vi "LAX100.vi"() -> ()   [LabVIEW 2015]
uses:
  <vilib>/Instr/_visa.llb/VISA Configure Serial Port (Instr).vi
panel:
  out "Serial Settings:Number of Bytes at Serial Port":u32
  out "error out 4":errorcluster
  out "error out":errorcluster
  out "error out 3":errorcluster
  out "VISA resource name out":refnum<visa-resource-name>
  in  "error out 2":errorcluster
  out "read buffer":string
  in  "stop":bool
  out "CMD":string
  in  "shutter":bool
  in  "power":bool
  in  "Intensity":dbl
  # "LAX-C100"
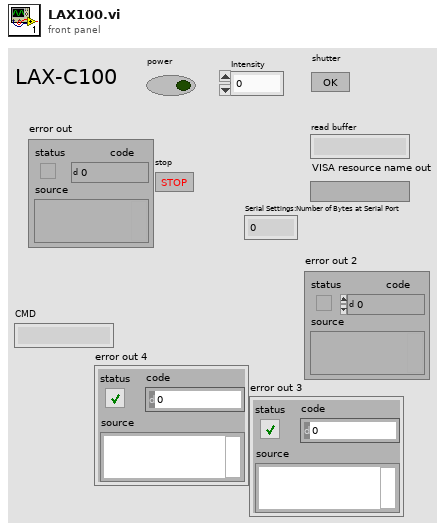
[diagram p1: front panel]
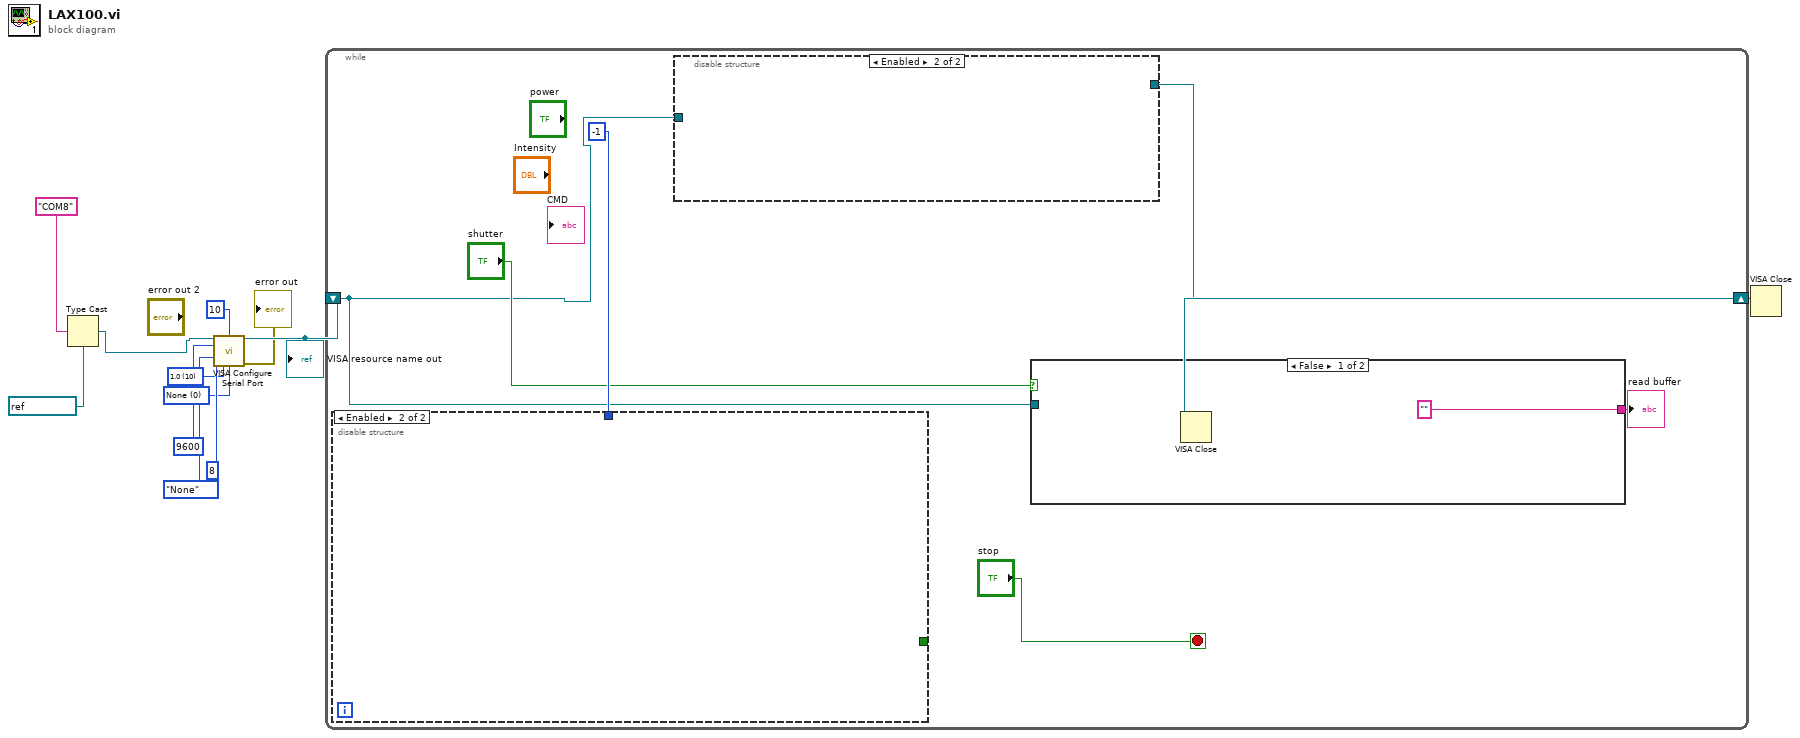
[diagram p0: block diagram]
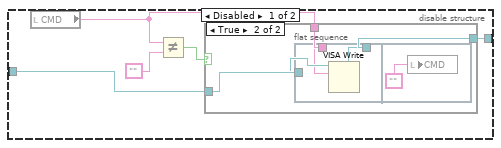
[diagram p2: hidden frame]
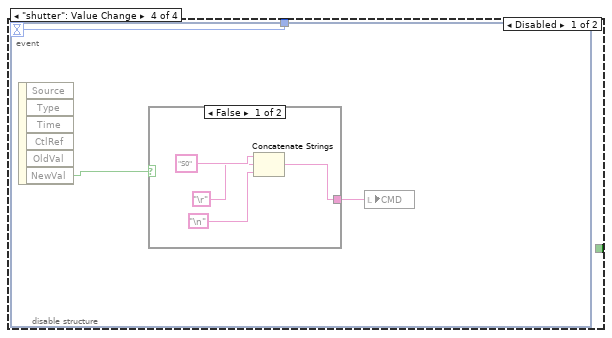
[diagram p4: hidden frame]
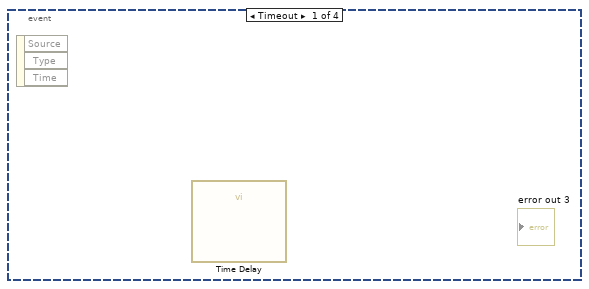
[diagram p5: hidden frame]
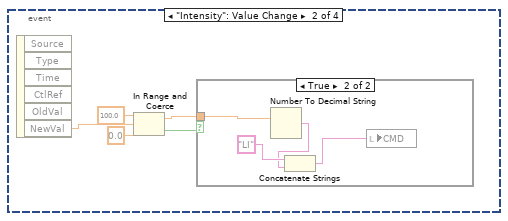
[diagram p6: hidden frame]
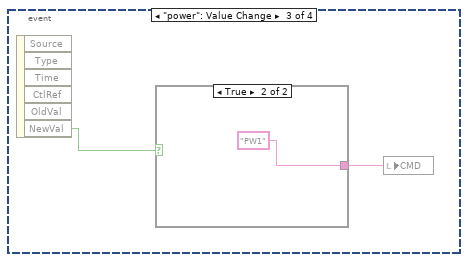
[diagram p8: hidden frame]
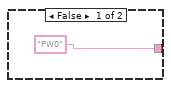
[diagram p9: hidden frame]
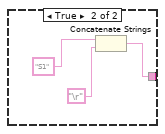
[diagram p10: hidden frame]
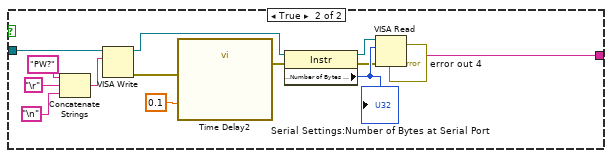
[diagram p11: hidden frame]
diagram:
  w6 = u16 0 items=["None", "XON/XOFF", "RTS/CTS", "XON/XOFF & RTS/CTS", "DTR/DSR", "XON/XOFF & DTR/DSR"] ("flow control (0:none)")
  w7 = u16 10 items=["1.0"=10, "1.5"=15, "2.0"=20] ("stop bits (10: 1 bit)")
  n1 = Type Cast(type=refnum<visa-resource-name> "COM12" ("VISA resource name"), x="COM8") -> (*(type *) &x=w2:refnum<visa-resource-name>)
  n2 = call-poly "VISA Configure Serial Port"("VISA resource name"=w2, "termination char\n(0xA = '\\n' = LF)"=u8 10 ("termination char\n(0xA = '\\n' = LF)"), "baud rate (9600)"=u32 9600, "data bits (8)"=u16 8, "parity (0:none)"=enum16{"None", "Odd", "Even", "Mark", "Space"}."None", "stop bits (10: 1 bit)"=w7, "flow control (0:none)"=w6) -> ("VISA resource name out"=w9:refnum<visa-resource-name>, "error out"=→"error out":errorcluster)  [unwired: 7 in]
  "VISA resource name out" <- w9
  n3 = while {
    shift-right: [w17] -> w8
    shift-left: w9 -> [w15]
    stop <- "stop" stop-if-true
    n4 = disable-structure shown="Enabled" {
      disable-tunnel: _ -> [w32 _]
      disable-tunnel: -1 -> [w31 _]
      frame Disabled {
        n5 = event shown="[3] \"shutter\": Value Change" {
          selector: _ -> [_ _ _ _]
          dyn-events: _ -> [_ _ _ _]
          timeout: w31 -> [_ _ _ _]
          event Timeout {
            n6 = event-data() -> ()  [unwired: 1 in, 3 out]
            n7 = call "Time Delay"() -> ()  [unwired: 11 in, 1 out]
          }
          event "Intensity": Value Change {
            n8 = event-data() -> ("NewVal"=w37:dbl)  [unwired: 1 in, 5 out]
            n9 = In Range and Coerce(upper limit=100.0, x=w37, lower limit=0.0) -> (coerced(x)=w33:dbl, In Range?=w34:bool)
            n10 = case shown="True" w34 {
              tunnel: w33 -> [_ w41]
              frame False {
              }
              frame True {
                n11 = Number To Decimal String(number=w41) -> (decimal integer string=w39:string)  [unwired: 1 in]
                n12 = Concatenate Strings("LI", w39) -> (w38:string)
                n13 = local write "CMD"(w38) -> ()
              }
            }
          }
          event "power": Value Change {
            n14 = event-data() -> ("NewVal"=w43:bool)  [unwired: 1 in, 5 out]
            n15 = case shown="True" w43 {
              tunnel: ["PW0" "PW1"] -> w42
              frame False {
              }
              frame True {
              }
            }
            n16 = local write "CMD"(w42) -> ()
          }
          event "shutter": Value Change {
            n17 = event-data() -> ("NewVal"=w47:bool)  [unwired: 1 in, 5 out]
            n18 = case shown="False" w47 {
              tunnel: [w50 w52] -> w46
              frame False {
                n19 = Concatenate Strings("S0", "\r", "\n") -> (w50:string)
              }
              frame True {
                n20 = Concatenate Strings("S1", "\r") -> (w52:string)
              }
            }
            n21 = local write "CMD"(w46) -> ()
          }
        }
      }
      frame Enabled {
      }
    }
    n22 = disable-structure shown="Enabled" {
      disable-tunnel: [w20 _] -> w17
      disable-tunnel: w15 -> [w19 _]
      frame Disabled {
        n23 = local read "CMD"() -> (w23:string)
        n24 = Not Equal?(x=w23, y="") -> (x != y?=w22:bool)
        n25 = case shown="True" w22 {
          tunnel: [_ w26] -> w20
          tunnel: w23 -> [_ w25]
          tunnel: w19 -> [_ w24]
          frame False {
          }
          frame True {
            n26 = flat-sequence {
              tunnel: [w29] -> w26
              tunnel: w24 -> [w28]
              tunnel: w25 -> [w27]
              frame #0 {
                n27 = VISA Write(VISA resource name=w28, write buffer=w27) -> (VISA resource name out=w29:refnum<visa-resource-name>)  [unwired: 1 in, 2 out]
              }
              frame #1 {
                n28 = local write "CMD"("") -> ()
              }
            }
          }
        }
      }
      frame Enabled {
      }
    }
    n29 = case shown="False" "shutter" {
      tunnel: w15 -> [_ w66]
      tunnel: ["" ("read buffer") w58] -> w14
      frame False {
      }
      frame True {
        n30 = Concatenate Strings("PW?", "\r", "\n") -> (w67:string)
        n31 = VISA Write(VISA resource name=w66, write buffer=w67) -> (VISA resource name out=w62:refnum<visa-resource-name>, error out=w65:errorcluster)  [unwired: 1 in, 1 out]
        n32 = call "Time Delay2"("error in (no error)"=w65, "Delay Time (s)"=0.1) -> ("error out"=w63:errorcluster)  [unwired: 9 in]
        n33 = property class="Instr"(reference=w62, error in=w63) -> (reference out=w61:refnum<visa-resource-name>, error out=w59:errorcluster, "Serial Settings:Number of Bytes at Serial Port"=w60:u32)
        "Serial Settings:Number of Bytes at Serial Port" <- w60
        n34 = VISA Read(VISA resource name=w61, byte count=w60, error in (no error)=w59) -> (read buffer=w58:string, error out=→"error out 4":errorcluster)  [unwired: 2 out]
      }
    }
    "read buffer" <- w14
  }
  n35 = VISA Close(VISA resource name=w8) -> ()  [unwired: 1 in, 1 out]
  n36 = VISA Close(VISA resource name=w8) -> ()  [unwired: 1 in, 1 out]
